vi "get DT.vi"(6 "Controls[]":refnum<vi>[](array[refnum]), 9 "variante?":bool, 10 "variante":string, 11 "Modello":string) -> (1 "tipo accoppiamento":i32, 2 "tipo alternatore":i32, 3 "tipo fissaggio":i32, 4 "ricetta":string)   [LabVIEW 2014]
uses:
  <vilib>/addons/database/Connection.llb/DB Tools Open Connec (String).vi
  <vilib>/addons/database/NI_Database_API.lvlib
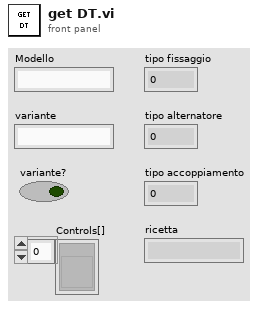
[diagram p1: front panel]
types:
  T1 = typedef "NI_Database_API.lvlib/Conn ObjectReference.ctl" = refnum<k1>
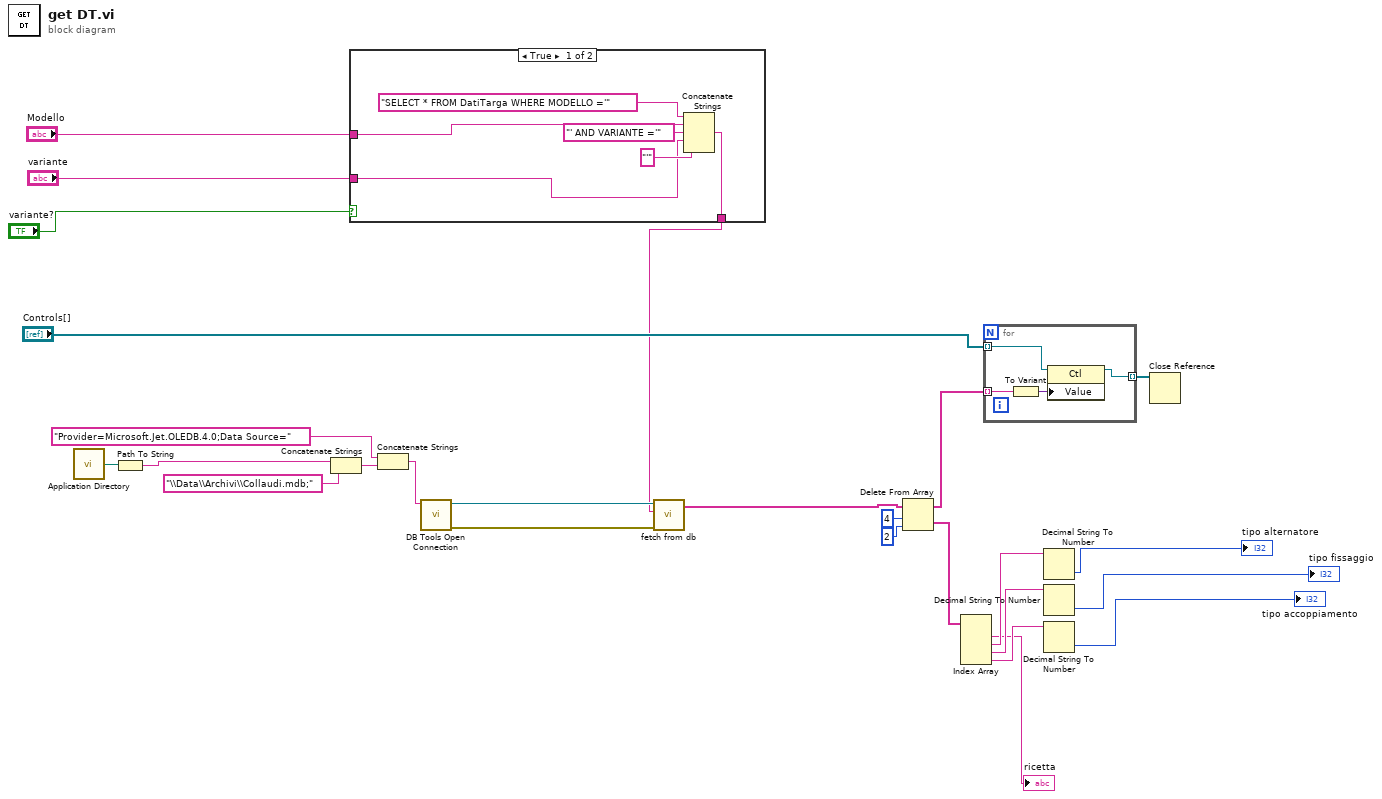
[diagram p0: block diagram]
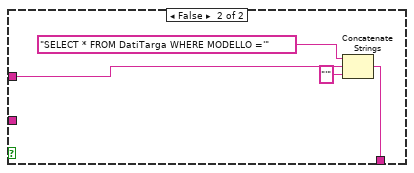
[diagram p2: hidden frame]
diagram:
  n1 = call <vilib>:"Application Directory.vi"() -> ("Application Directory"=w15:path)
  n2 = Path To String(path=w15) -> (string=w16:string)
  n3 = Concatenate Strings(w16, "\\Data\\Archivi\\Collaudi.mdb;" ("string")) -> (w14:string)
  n4 = case shown="True" "variante?" {
    tunnel: [w29 w35] -> w2
    tunnel: "Modello" -> [w28 w33]
    tunnel: "variante" -> [w27 _]
    frame True {
      n5 = Concatenate Strings("SELECT * FROM DatiTarga WHERE MODELLO ='" ("SQL query"), w28, "' AND VARIANTE ='" ("string"), w27, "'" ("string")) -> (w29:string)
    }
    frame False {
      n6 = Concatenate Strings("SELECT * FROM DatiTarga WHERE MODELLO ='" ("SQL query"), w33, "'" ("string")) -> (w35:string)
    }
  }
  n7 = Concatenate Strings("Provider=Microsoft.Jet.OLEDB.4.0;Data Source=" ("string"), w14) -> (w13:string)
  n8 = call-poly <vilib>:"DB Tools Open Connection.vi"("connection information"=w13) -> ("error out"=w1:errorcluster, "connection reference"=w17:T1)  [unwired: 7 in]
  n9 = call "fetch from db.vi"("error in (no error)"=w1, "istruzione select from"=w2, "Refnum in"=w17) -> ("data"=w3:string[])  [unwired: 8 in]
  n10 = Delete From Array(array=w3, length=4, index=2) -> (deleted portion=w9:string[], array with subset deleted=w7:string[])
  n11 = Index Array(array=w9) -> (element #1=→"ricetta":string, element #2=w19:string, element #3=w21:string, element #4=w23:string)  [unwired: 4 in]
  n12 = for {
    tunnel: "Controls[]" -> [w39] mode=indexing
    tunnel: w7 -> [w38] mode=indexing
    tunnel: [w37] -> w18 mode=indexing
    n13 = To Variant(anything=w38) -> (Variant=w40:variant)
    n14 = property class="Ctl"(reference=w39, "Value"=w40) -> (reference out=w37:refnum<vi>)  [unwired: 1 in, 1 out]
  }
  n15 = Decimal String To Number(string=w19) -> (number=→"tipo alternatore":i32)  [unwired: 2 in, 1 out]
  n16 = Decimal String To Number(string=w21) -> (number=→"tipo fissaggio":i32)  [unwired: 2 in, 1 out]
  n17 = Decimal String To Number(string=w23) -> (number=→"tipo accoppiamento":i32)  [unwired: 2 in, 1 out]
  n18 = Close Reference(reference=w18) -> ()  [unwired: 1 in, 1 out]
